vi "Pickup State Machine.vi"   [LabVIEW 2013]
uses:
  typedefs/fg_typedef.ctl
  typedefs/State Machine/subStates.ctl
  typedefs/DevRef Type.ctl
panel:
  # "A State Machine to Handle Pickup for Passing"
types:
  T1 = typedef "subStates.ctl" = enum16{"null", "wait", "driver control", "auto", "manual override", "hold position", "rotate", "pickup", "pass", "recover pass", "load", "goto shoot", "shoot high goal", "shoot low goal", "cancel arm", "cancel shooter", "end", "test"}
  T2 = typedef "fg_typedef.ctl" = enum16{"Get", "Set"}
  T3 = typedef "DevRef Type.ctl" = enum16{"Shooter Solenoid", "Latch Solenoid", "Right Up Sensor", "Right Down Sensor", "Hold Sensor", "Arm Encoder"}
  T4 = typedef "WPI_DigitalInputDevRef.ctl" = cluster{"DevStatus":errorcluster, "DIO Channel":T5, "Digital Module":T6}
  T5 = typedef "FPGA_DIOChannel.ctl" = enum8{"DIO 1", "DIO 2", "DIO 3", "DIO 4", "DIO 5", "DIO 6", "DIO 7", "DIO 8", "DIO 9", "DIO 10", "DIO 11", "DIO 12", "DIO 13", "DIO 14", "Invalid"}
  T6 = typedef "FPGA_TypedefDigitalModule.ctl" = enum16{"Digital Module 1", "Digital Module 2"}
  T7 = typedef "WPI_EncoderDevRef.ctl" = cluster{"DevStatus":errorcluster, "EncoderIndex":T8, "CounterIndex":T9, "DistancePerCount":dbl, "Decoding Type":T10}
  T8 = typedef "FPGA_EncoderIdx.ctl" = enum8{"Enc 0", "Enc 1", "Enc 2", "Enc 3", "Invalid"}
  T9 = typedef "FPGA_CounterCtrSystemIndex.ctl" = enum8{"Ctr 0", "Ctr 1", "Ctr 2", "Ctr 3", "Ctr 4", "Ctr 5", "Ctr 6", "Ctr 7", "Invalid"}
  T10 = typedef "WPI_EncoderType.ctl" = enum16{"1x", "2x", "4x"}
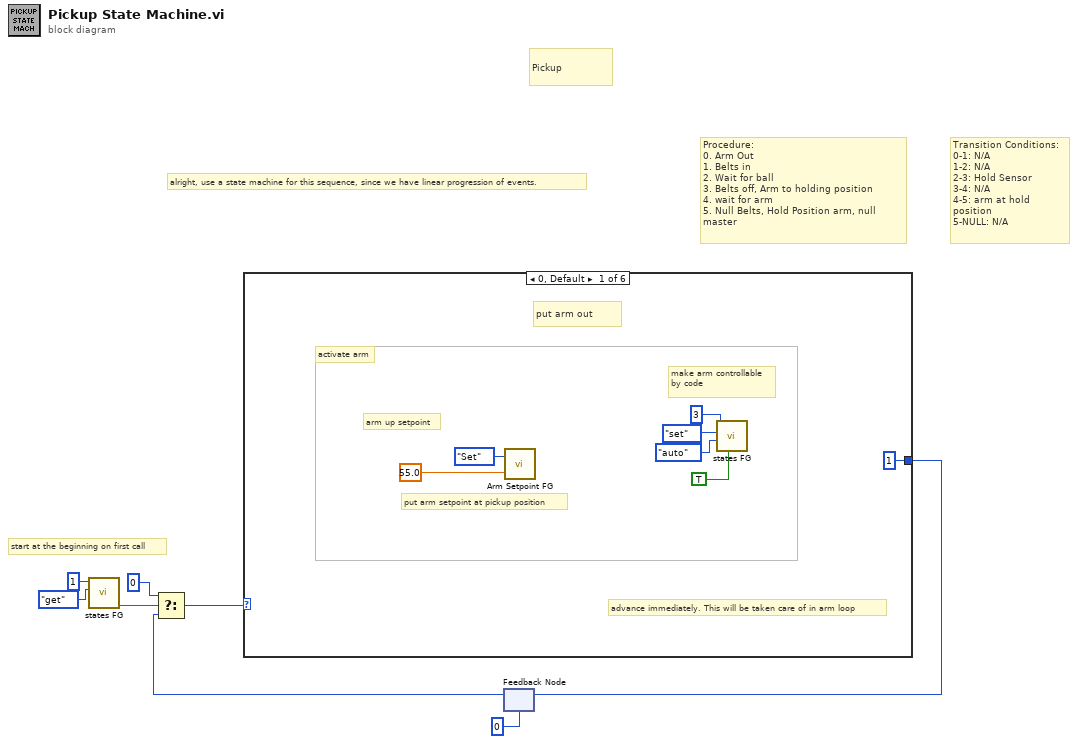
[diagram p0: block diagram]
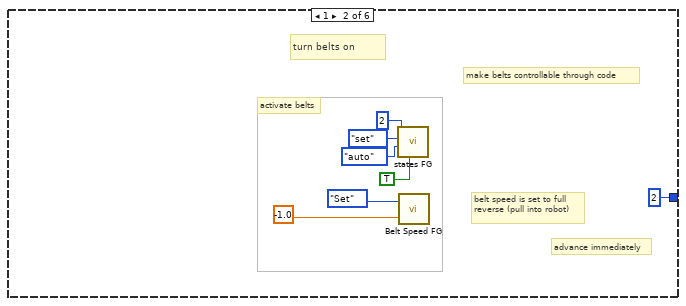
[diagram p2: hidden frame]
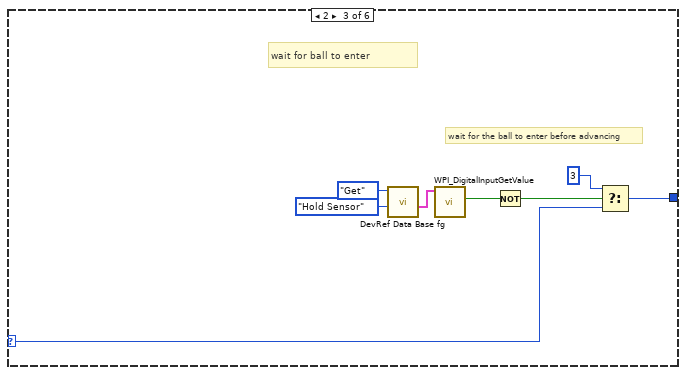
[diagram p3: hidden frame]
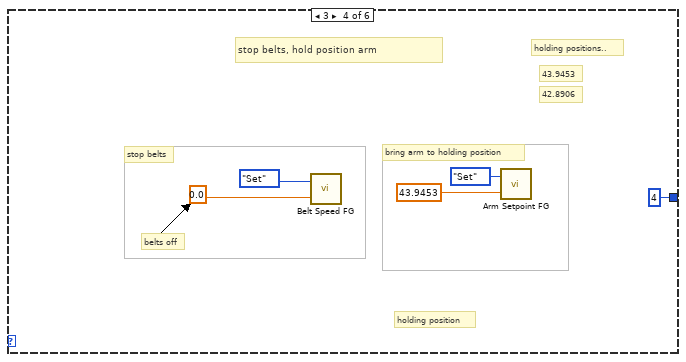
[diagram p4: hidden frame]
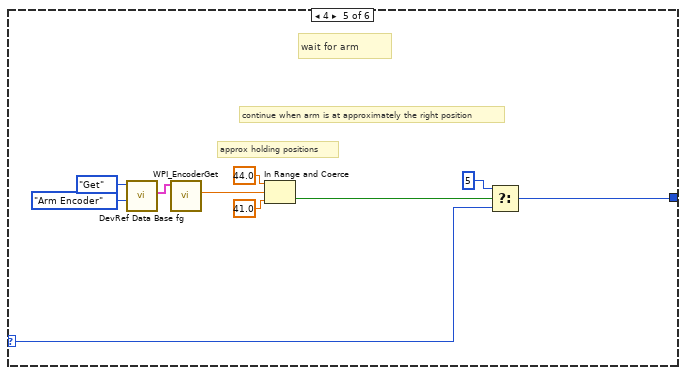
[diagram p5: hidden frame]
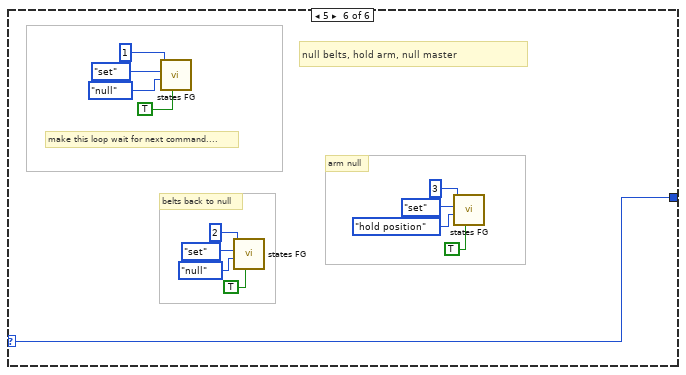
[diagram p6: hidden frame]
diagram:
  # "Transition Conditions:\n0-1: N/A\n1-2: N/A\n2-3: Hold Sensor \n3-4: N/A\n4-5: arm at hold position\n5-NULL: N/A"
  # "start at the beginning on first call"
  # "Pickup"
  # "Procedure: \n0. Arm Out\n1. Belts in\n2. Wait for ball\n3. Belts off, Arm to holding position\n4. wait for arm\n5. Null Belts, Hold Position arm, null master"
  # "alright, use a state machine for this sequence, since we have linear progression of events."
  n1 = call "states FG.vi"("menu (get)"=enum16{"set", "get"}."get", "Loop ID"=1) -> ("first call?"=w1:bool)  [unwired: 6 in, 3 out]
  n2 = feedback #1(u8 0) -> (w2:u8)
  n3 = Select(t=u8 0, s=w1, f=w2) -> (s? t:f=w4:u8)
  n4 = case shown="0, Default" w4 {
    selector: w4 -> [_ _ w29 _ w38 w50]
    tunnel: [u8 1 ("t") u8 2 ("t") w28 u8 4 ("t") w41 w50] -> w7
    frame 0, Default {
      # "arm up setpoint"
      # "put arm setpoint at pickup position"
      # "activate arm"
      # "make arm controllable\nby code"
      # "advance immediately. This will be taken care of in arm loop"
      # "put arm out"
      n5 = call "Arm Setpoint FG.vi"("Setpoint In"=55.0, "Menu"=fg_typedef."Set") -> ()  [unwired: 1 out]
      n6 = call "states FG.vi"("exit in"=TRUE, "subState in"=subStates."auto", "menu (get)"=enum16{"set", "get"}."set", "Loop ID"=3) -> ()  [unwired: 4 in, 4 out]
    }
    frame 1 {
      # "advance immediately"
      # "belt speed is set to full\nreverse (pull into robot)"
      # "make belts controllable through code"
      # "activate belts"
      # "turn belts on"
      n7 = call "states FG.vi"("exit in"=TRUE, "subState in"=subStates."auto", "menu (get)"=enum16{"set", "get"}."set", "Loop ID"=2) -> ()  [unwired: 4 in, 4 out]
      n8 = call "Belt Speed FG.vi"("Speed In"=-1.0 ("Setpoint In"), "Menu"=fg_typedef."Set") -> ()  [unwired: 1 out]
    }
    frame 2 {
      # "wait for ball to enter"
      # "wait for the ball to enter before advancing"
      n9 = call "DevRef Data Base fg.vi"("DevRef to Get"=DevRef_Type."Hold Sensor", "Menu"=fg_typedef."Get") -> ("Selected Sensor"=w27:T4)  [unwired: 1 in, 8 out]
      n10 = call <vilib>:"WPI_DigitalInputGetValue.vi"("DigitalInputDevRef"=w27) -> ("Value"=w30:bool)  [unwired: 8 in, 2 out]
      n11 = Not(x=w30) -> (.not. x?=w25:bool)
      n12 = Select(t=u8 3, s=w25, f=w29) -> (s? t:f=w28:u8)
    }
    frame 3 {
      # "holding position"
      # "stop belts, hold position arm"
      # "42.8906"
      # "holding positions.."
      # "43.9453"
      # "stop belts"
      # "bring arm to holding position"
      # "belts off"
      n13 = call "Belt Speed FG.vi"("Speed In"=0.0 ("Setpoint In"), "Menu"=fg_typedef."Set") -> ()  [unwired: 1 out]
      n14 = call "Arm Setpoint FG.vi"("Setpoint In"=43.9453, "Menu"=fg_typedef."Set") -> ()  [unwired: 1 out]
    }
    frame 4 {
      # "approx holding positions"
      # "wait for arm"
      # "continue when arm is at approximately the right position"
      n15 = call "DevRef Data Base fg.vi"("DevRef to Get"=DevRef_Type."Arm Encoder", "Menu"=fg_typedef."Get") -> ("Selected Encoder"=w45:T7)  [unwired: 1 in, 8 out]
      n16 = call <vilib>:"WPI_EncoderGet.vi"("EncoderDevRef"=w45) -> ("Distance"=w44:dbl)  [unwired: 5 in, 5 out]
      n17 = In Range and Coerce(upper limit=44.0, x=w44, lower limit=41.0 ("upper limit")) -> (In Range?=w40:bool)  [unwired: 1 out]
      n18 = Select(t=u8 5, s=w40, f=w38) -> (s? t:f=w41:u8)
    }
    frame 5 {
      # "belts back to null"
      # "make this loop wait for next command...."
      # "arm null"
      # "null belts, hold arm, null master"
      n19 = call "states FG.vi"("exit in"=TRUE, "subState in"=subStates."null", "menu (get)"=enum16{"set", "get"}."set", "Loop ID"=1) -> ()  [unwired: 4 in, 4 out]
      n20 = call "states FG.vi"("exit in"=TRUE, "subState in"=subStates."null", "menu (get)"=enum16{"set", "get"}."set", "Loop ID"=2) -> ()  [unwired: 4 in, 4 out]
      n21 = call "states FG.vi"("exit in"=TRUE, "subState in"=subStates."hold position", "menu (get)"=enum16{"set", "get"}."set", "Loop ID"=3) -> ()  [unwired: 4 in, 4 out]
    }
  }
  n22 = feedback-in #1(w7) -> ()
